vi "Printing test.vi"() -> ()   [LabVIEW 2012]
uses:
  <vilib>/Utility/NIReport.llb/NI_report.lvclass
  <vilib>/Utility/NIReport.llb/Append Image to Report (path wrap).vi
panel:
  in  "report type":T1(ring)=enum."HTML"
  in  "Print":bool
  in  "stop":bool
  in  "Path":path=path "C:/Users/Public/AutoCal/Calibration Q1 Report Pg 1 of 2 - 140313 2130.jpg"
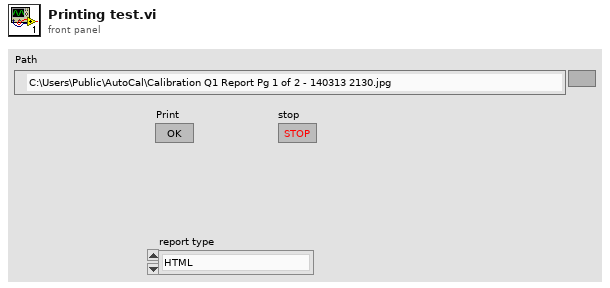
[diagram p1: front panel]
types:
  T1 = enum16{"Standard Report", "HTML", "Word", "Excel"}
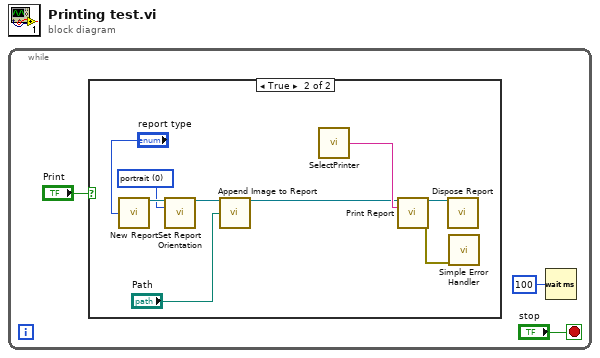
[diagram p0: block diagram]
diagram:
  n1 = while {
    stop <- "stop" stop-if-true
    n2 = case shown="True" "Print" {
      frame False {
      }
      frame True {
        w9 = 0 items=["portrait", "landscape"] ("orientation (portrait)")
        n3 = call <vilib>:"New Report.vi"("report type"="report type") -> ("report out"=w10:refnum<class "NI_report.lvclass">)  [unwired: 13 in, 1 out]
        n4 = call-dynamic "Set Report Orientation.vi"("report in"=w10, "orientation (portrait)"=w9) -> ("report out"=w5:refnum<class "NI_report.lvclass">)  [unwired: 12 in, 1 out]
        n5 = call-poly <vilib>:"Append Image to Report.vi"("report in"=w5, "path or URL of image"="Path") -> ("report out"=w4:refnum<class "NI_report.lvclass">)  [unwired: 10 in, 3 out]
        n6 = call "SelectPrinter.vi"() -> ("ChosenPrinter"=w6:string)
        n7 = call-dynamic "Print Report.vi"("report in"=w4, "printer name (default)"=w6) -> ("report out"=w11:refnum<class "NI_report.lvclass">, "error out"=w7:errorcluster)  [unwired: 12 in]
        n8 = call-dynamic "Dispose Report.vi"("report in"=w11) -> ()  [unwired: 14 in, 1 out]
        n9 = call <vilib>:"Simple Error Handler.vi"("error in (no error)"=w7) -> ()  [unwired: 4 in, 5 out]
      }
    }
    n10 = Wait (ms)(milliseconds to wait=u32 100) -> ()  [unwired: 1 out]
  }
